vi "Keithley 6517A LTCC Single Read.vi"(8 "error in":T1, 9 "Read Displays":bool=TRUE, 11 "GPIB address":string="1:27") -> (0 "error out":T1, 1 "time and date stamp":string="0", 2 "Time":string="03:56:06.00", 3 "measurement":dbl format="%.6e", 4 "secondary display":string="0\n", 5 "units":string="0", 6 "reading #":dbl, 7 "primary display":string="0\n")   [LabVIEW 2024]
doc: "This VI takes a single reading from the 6517. The data returned includes the reading, timestamp, units, and reading#."
panel:
  out "Raw Readback":string="0\n"
  # "(A)"
  # "ON\nOFF"
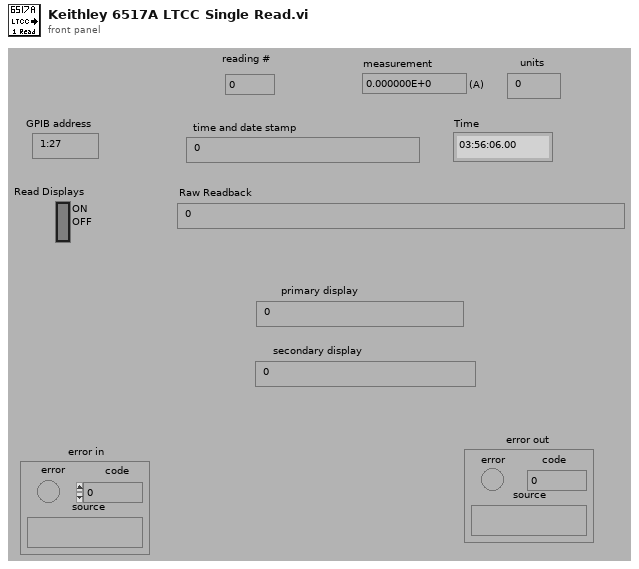
[diagram p1: front panel]
types:
  T1 = cluster{"error":bool, "code":i32, "source":string}
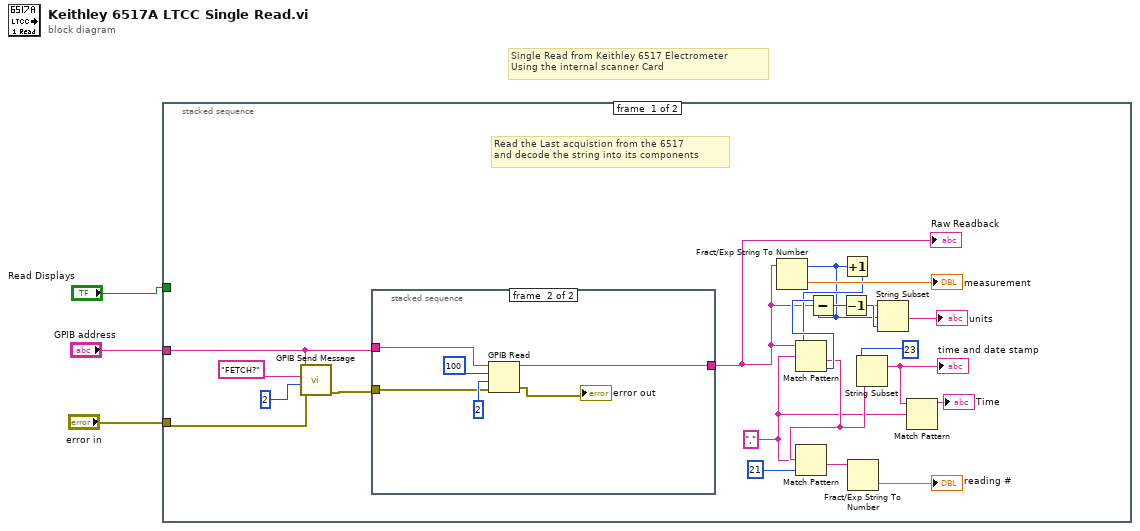
[diagram p0: block diagram]
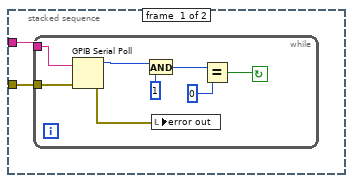
[diagram p2: hidden frame]
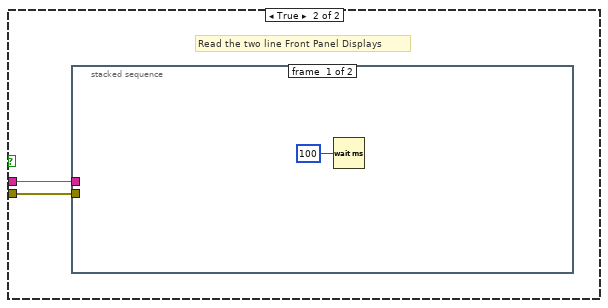
[diagram p4: hidden frame]
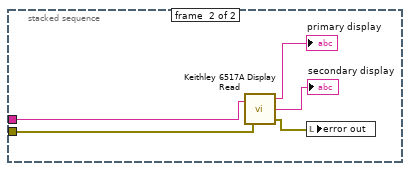
[diagram p5: hidden frame]
diagram:
  # "Single Read from Keithley 6517 Electrometer \nUsing the internal scanner Card"
  n1 = stacked-sequence {
    tunnel: "GPIB address" -> [w9 w42]
    tunnel: "error in" -> [w7 w41]
    tunnel: "Read Displays" -> [_ w43]
    frame #0 {
      w6 = ","
      # "Read the Last acquistion from the 6517\nand decode the string into its components"
      n2 = call "GPIB Send Message.vi"("address string"=w9, "write buffer"="FETCH?", "write mode (set END:0)"=2, "error in"=w7) -> ("error out"=w10:T1)  [unwired: 3 in, 2 out]
      n3 = stacked-sequence {
        tunnel: [_ w40] -> w8
        tunnel: w10 -> [w25 w37]
        tunnel: w9 -> [w26 w36]
        frame #0 {
          n4 = while {
            tunnel: w26 -> [w29]
            tunnel: w25 -> [w28]
            stop <- w33 continue-if-true
            n5 = GPIB Serial Poll(0:w29, 1:w28) -> (2:w32:i16, 4:w27:errorcluster)  [unwired: 1 out]
            n6 = And(x=w32, y=1) -> (x .and. y?=w30:i32)
            n7 = local write "error out"(w27) -> ()
            n8 = Equal?(x=w30, y=0) -> (x = y?=w33:bool)
          }
        }
        frame #1 {
          n9 = GPIB Read(0:w36, 1:100, 2:2, 3:w37) -> (5:w40:string, 7:→"error out":errorcluster)  [unwired: 1 in, 1 out]
        }
      }
      "Raw Readback" <- w8
      n10 = Fract/Exp String To Number(string=w8) -> (offset past number=w13:i32, number=→"measurement":dbl)  [unwired: 3 in]
      n11 = Increment(x=w13) -> (x+1=w14:i32)
      n12 = Match Pattern(string=w8, regular expression=w6, offset (0)=w14) -> (after substring=w16:string, offset past match=w20:i32)  [unwired: 2 out]
      n13 = Match Pattern(string=w16, regular expression=w6, offset (0)=21) -> (after substring=w21:string)  [unwired: 3 out]
      n14 = Subtract(x=w20, y=w13) -> (x-y=w18:i32)
      n15 = Decrement(x=w18) -> (x-1=w19:i32)
      n16 = Fract/Exp String To Number(string=w21) -> (number=→"reading #":dbl)  [unwired: 3 in, 1 out]
      n17 = String Subset(string=w16, length (rest)=23) -> (substring=w5:string)  [unwired: 1 in]
      "time and date stamp" <- w5
      n18 = String Subset(string=w8, offset (0)=w13, length (rest)=w19) -> (substring=→"units":string)
      n19 = Match Pattern(string=w5, regular expression=w6) -> (before substring=→"Time":string)  [unwired: 1 in, 3 out]
    }
    frame #1 {
      n20 = case shown="False" w43 {
        tunnel: w42 -> [_ w45]
        tunnel: w41 -> [_ w44]
        frame False {
        }
        frame True {
          # "Read the two line Front Panel Displays"
          n21 = stacked-sequence {
            tunnel: w45 -> [_ w51]
            tunnel: w44 -> [_ w50]
            frame #0 {
              n22 = Wait (ms)(milliseconds to wait=u32 100) -> ()  [unwired: 1 out]
            }
            frame #1 {
              n23 = call "Keithley 6517A Display Read.vi"("GPIB address"=w51, "error in"=w50) -> ("primary display"=→"primary display":string, "secondary display"=→"secondary display":string, "error out"=w47:T1)
              n24 = local write "error out"(w47) -> ()
            }
          }
        }
      }
    }
  }
